vi "AMX-电源头正面标签1检测参数读取.vi"(7 "error in (no error)":errorcluster caption="错误输入（无错误）", 10 "基路径":path) -> (0 "error out":errorcluster caption="错误输出", 1 "CCD1参数":T5={"Rectangle"={"Left"=1952, "Top"=146, "Right"=370, "Bottom"=2690, "Rotation"=45.0}, "Angle (degrees) "=90.0, "long"=150.0, "abgek"=-90.0, "Color"=16711680, "left threshold"=0.0, "Rectangle right"={"Left"=1952, "Top"=1596, "Right"=570, "Bottom"=2690, "Rotation"=45.0}, "long right"=150.0, "abgek right"=90.0, "Color 2"=16711680, "right threshold"=0.0, "left"=0.0, "right"=0.0, "Settings (Big)"={"Extraction Mode"=0, "Edge Threshold"=17, "Edge Filter Size"=1, "Min Length"=36, "Row Search Step Size"=13, "Col Search Step Size"=13, "Max Endpoint Gap"=10, "Closed"=FALSE, "Subpixel"=TRUE}, "Clamp Settings (Big)"={"Angle "=10.0, "Edge Polarity"={"Start"=0, "End"=0}}, " Settings top"={"Extraction Mode"=0, "Edge Threshold"=18, "Edge Filter Size"=1, "Min Length"=36, "Row Search Step Size"=64, "Col Search Step Size"=64, "Max Endpoint Gap"=10, "Closed"=FALSE, "Subpixel"=TRUE}, "Clamp Settings top "={"Angle "=10.0, "Edge Polarity"={"Start"=0, "End"=0}}, "Sub-Pixel Accuracy "=TRUE, "Threshold Parameters"={"Level Type"=enum."Absolute Value", "Threshold Level"=127, "Hysteresis"=2}, "Process "=enum."Get First + Last Edge", "Threshold Parameters 2"={"Level Type"=enum."Absolute Value", "Threshold Level"=127, "Hysteresis"=2}} {"Clamp Settings top"."Edge Polarity"."Start" items=["Any", "Rising", "Falling"]; "Clamp Settings top"."Edge Polarity"."End" items=["Any", "Rising", "Falling"]; "Settings top"."Extraction Mode" items=["Normal", "Uniform Regions"]; "Settings top"."Edge Filter Size" items=["Fine", "Normal", "Contour Tracing"]; "Settings top"."Max Endpoint Gap" min=0; "Settings top"."Col Search Step Size" min=1 max=255 step=1; "Settings top"."Row Search Step Size" min=1 max=255 step=1; "Settings top"."Min Length" min=0; "Settings top"."Edge Threshold" min=1 max=350 step=1; "Clamp Settings (Big)"."Edge Polarity"."Start" items=["Any", "Rising", "Falling"]; "Clamp Settings (Big)"."Edge Polarity"."End" items=["Any", "Rising", "Falling"]; "Settings (Big)"."Extraction Mode" items=["Normal", "Uniform Regions"]; "Settings (Big)"."Edge Filter Size" items=["Fine", "Normal", "Contour Tracing"]; "Settings (Big)"."Max Endpoint Gap" min=0; "Settings (Big)"."Col Search Step Size" min=1 max=255 step=1; "Settings (Big)"."Row Search Step Size" min=1 max=255 step=1; "Settings (Big)"."Min Length" min=0; "Settings (Big)"."Edge Threshold" min=1 max=350 step=1; "Rectangle right"."Rotation" format="%.2f"; "Rectangle right"."Left" scale=0.0..1024.0; "Rectangle right"."Right" scale=0.0..1024.0; "Rectangle"."Rotation" format="%.2f"; "Rectangle"."Left" scale=0.0..1024.0; "Rectangle"."Right" scale=0.0..1024.0}, 2 "CCD1基础参数":T6={"IsNorImage"=TRUE, "Exposure Values"=100289, "ImagePath"=path "C:/Users/hedongpo/Desktop/514-hdp/Alignment Assemble System/Test Picture/B/3.bmp"} caption="参数界面" {"Exposure Values" scale=0.0..200000.0}, 3 "CCD1 ROI参数":T3={"Rectangle big CCD1"={"Left"=1952, "Top"=1596, "Right"=570, "Bottom"=2690, "Rotation"=45.0}, "Rectangle top CCD1 "={"Left"=1952, "Top"=1596, "Right"=570, "Bottom"=2690, "Rotation"=45.0}, "Line"={"Start X"=0, "Start Y"=0, "End X"=0, "End Y"=0}, "left line "=846.0, "right line"=1152.0} {"Line"."Start X" scale=0.0..1024.0; "Line"."End X" scale=0.0..1024.0; "Rectangle top CCD1"."Rotation" format="%.2f"; "Rectangle top CCD1"."Left" scale=0.0..1024.0; "Rectangle top CCD1"."Right" scale=0.0..1024.0; "Rectangle big CCD1"."Rotation" format="%.2f"; "Rectangle big CCD1"."Left" scale=0.0..1024.0; "Rectangle big CCD1"."Right" scale=0.0..1024.0})   [LabVIEW 2017]
uses:
  <vilib>/vision/Pattern Matching.llb/IMAQ Curve Parameters.ctl
  <vilib>/Utility/xml.llb/Read From XML File(string).vi
  Global System.vi
panel:
  # "箭头指示参数"
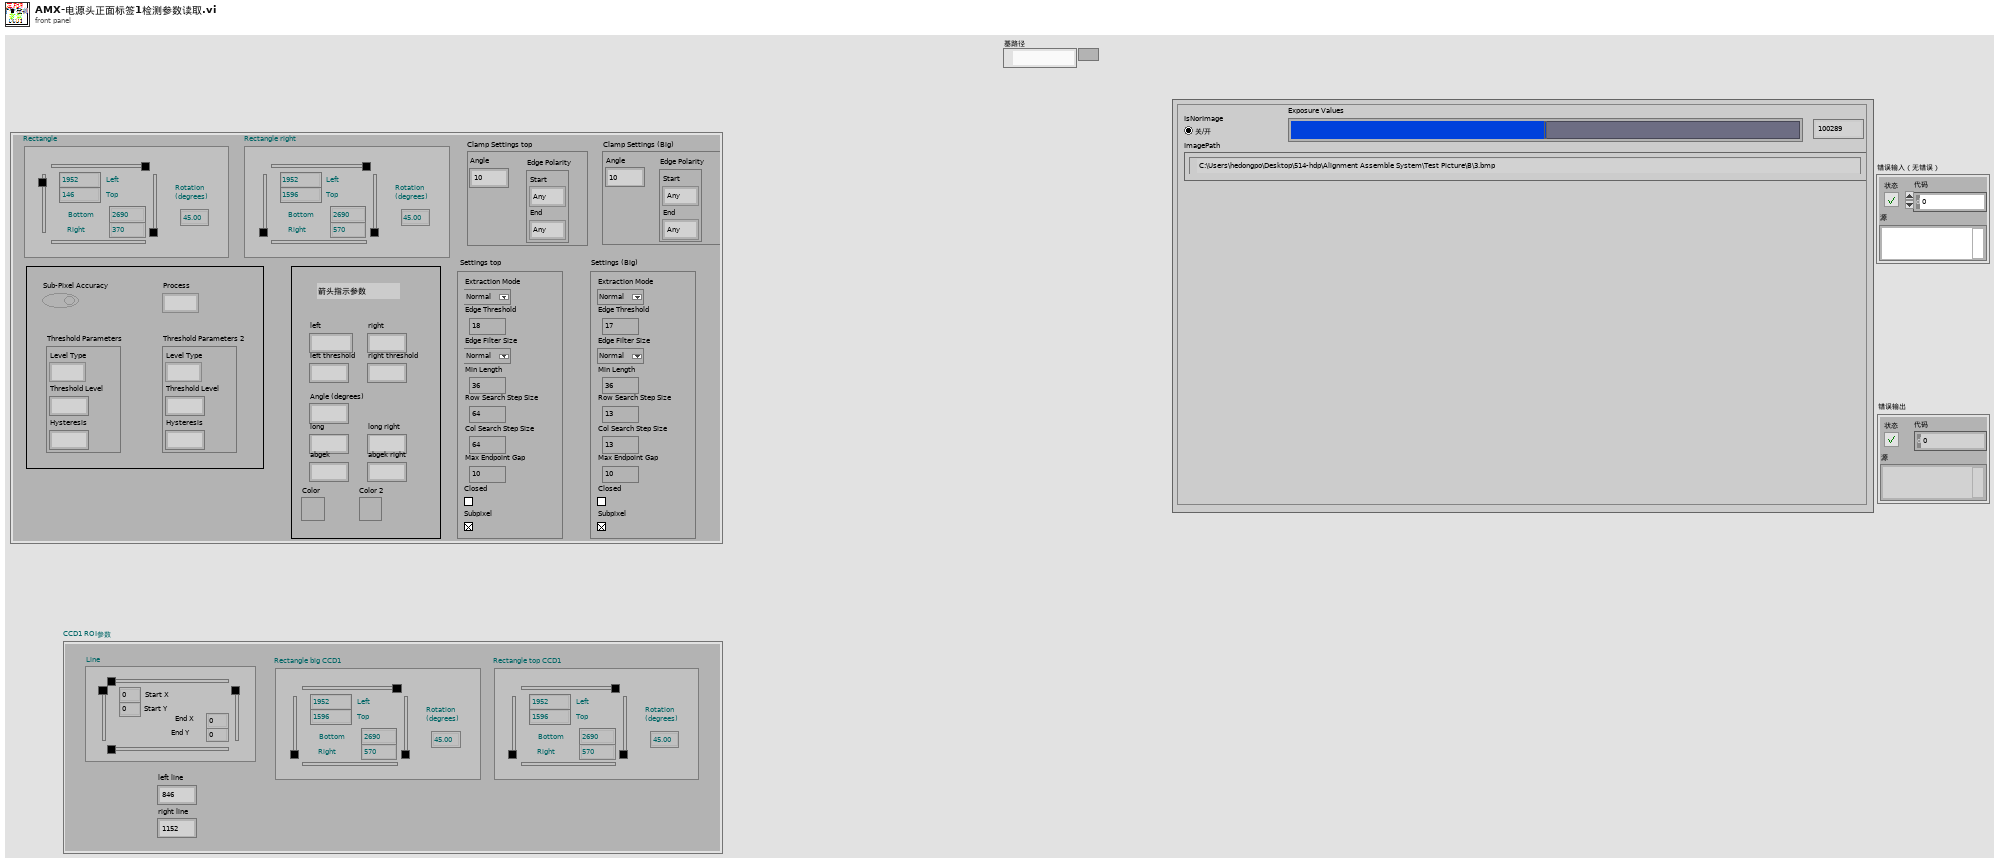
[diagram p1: front panel]
types:
  T1 = typedef "IMAQ Rectangle" = cluster{"Left":i32, "Top":i32, "Right":i32, "Bottom":i32, "Rotation":dbl}
  T2 = typedef "IMAQ Line" = cluster{"Start X":i32, "Start Y":i32, "End X":i32, "End Y":i32}
  T3 = cluster{"Rectangle big CCD1":T1, "Rectangle top CCD1 ":T1, "Line":T2, "left line ":dbl, "right line":dbl}
  T4 = typedef "IMAQ Curve Parameters.ctl" = cluster{"Extraction Mode":u32, "Edge Threshold":i32, "Edge Filter Size":u32, "Min Length":i32, "Row Search Step Size":i32, "Col Search Step Size":i32, "Max Endpoint Gap":i32, "Closed":bool, "Subpixel":bool}
  T5 = cluster{"Rectangle":T1, "Angle (degrees) ":sgl, "long":sgl, "abgek":dbl, "Color":u32, "left threshold":dbl, "Rectangle right":T1, "long right":sgl, "abgek right":dbl, "Color 2":u32, "right threshold":dbl, "left":dbl, "right":dbl, "Settings (Big)":T4, "Clamp Settings (Big)":cluster{"Angle ":dbl, "Edge Polarity":cluster{"Start":u32, "End":u32}}, " Settings top":T4, "Clamp Settings top ":cluster{"Angle ":dbl, "Edge Polarity":cluster{"Start":u32, "End":u32}}, "Sub-Pixel Accuracy ":bool, "Threshold Parameters":cluster{"Level Type":enum32{"Absolute Value", "Relative value"}, "Threshold Level":i32, "Hysteresis":i32}, "Process ":enum16{"Get First Edge", "Get First + Last Edge", "Get All Edges"}, "Threshold Parameters 2":cluster{"Level Type":enum32{"Absolute Value", "Relative value"}, "Threshold Level":i32, "Hysteresis":i32}}
  T6 = cluster{"IsNorImage":bool, "Exposure Values":u32, "ImagePath":path}
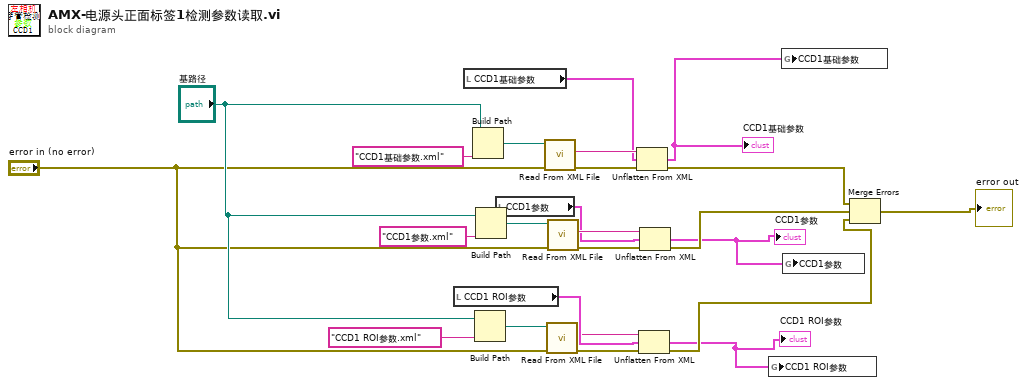
[diagram p0: block diagram]
diagram:
  n1 = local read "CCD1 ROI参数"() -> (w6:T3)
  n2 = local read "CCD1基础参数"() -> (w21:T6)
  n3 = Build Path(base path="基路径", name or relative path="CCD1基础参数.xml" ("名称或相对路径")) -> (appended path=w23:path)
  n4 = Build Path(base path="基路径", name or relative path="CCD1 ROI参数.xml" ("名称或相对路径")) -> (appended path=w3:path)
  n5 = Build Path(base path="基路径", name or relative path="CCD1参数.xml" ("名称或相对路径")) -> (appended path=w15:path)
  n6 = local read "CCD1参数"() -> (w11:T5)
  n7 = call-poly <vilib>:"Read From XML File.vi"("error in (no error)"="error in (no error)", "XML File Path"=w23) -> ("error out"=w20:errorcluster, "XML Elements"=w22:string)  [unwired: 7 in, 1 out]
  n8 = call-poly <vilib>:"Read From XML File.vi"("error in (no error)"="error in (no error)", "XML File Path"=w3) -> ("error out"=w5:errorcluster, "XML Elements"=w2:string)  [unwired: 7 in, 1 out]
  n9 = call-poly <vilib>:"Read From XML File.vi"("error in (no error)"="error in (no error)", "XML File Path"=w15) -> ("error out"=w13:errorcluster, "XML Elements"=w16:string)  [unwired: 7 in, 1 out]
  n10 = Unflatten From XML(xml string=w22, type=w21, error in (no error)=w20) -> (value=w18:T6, error out=w19:errorcluster)
  "CCD1基础参数" <- w18
  n11 = Unflatten From XML(xml string=w2, type=w6, error in (no error)=w5) -> (value=w1:T3, error out=w7:errorcluster)
  "CCD1 ROI参数" <- w1
  n12 = Unflatten From XML(xml string=w16, type=w11, error in (no error)=w13) -> (value=w10:T5, error out=w12:errorcluster)
  "CCD1参数" <- w10
  n13 = global write "Global System.vi" "CCD1 ROI参数"(w1) -> ()
  n14 = global write "Global System.vi" "CCD1基础参数"(w18) -> ()
  n15 = global write "Global System.vi" "CCD1参数"(w10) -> ()
  n16 = Merge Errors(w19, w12, w7) -> (→"error out":errorcluster)
